vi "Sig_Digital_GetAttributes.vi"(0 "reference in":refnum<class "Sig_Digital.lvclass">, 1 "return data? (T)":bool=TRUE, 5 "error in (no error)":errorcluster) -> (14 "reference out":refnum<class "Sig_Digital.lvclass">, 15 "attributes ref":T3, 16 "attributes":T1, 19 "error out":errorcluster)   [LabVIEW 2019]
doc: "Returns a reference and if wanted the actual data values of the attributes. This method is used by the subclasses to access parent attributes."
uses:
  protected/ObjectAttributes.ctl
  Sig_Digital.lvclass
  ObjectAttributesRef.ctl
  <vilib>/addons/_AddQ/G#Object/G#Object.lvclass
  D:/LabASF/LabASF/src/Signal_class/Signal.lvclass
  D:/LabASF/LabASF/src/Proccess_class/Proccess.lvclass
  TypeDef/Config_Digital.ctl
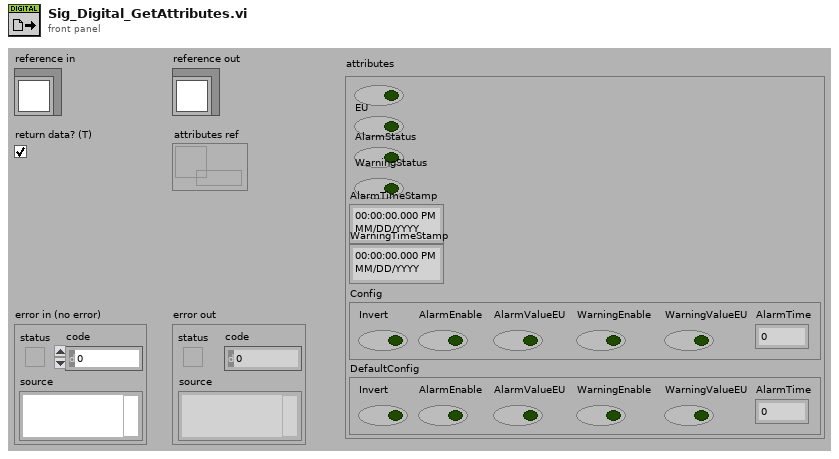
[diagram p1: front panel]
types:
  T1 = typedef "Sig_Digital.lvclass/ObjectAttributes.ctl" = cluster{"RAW":bool, "EU":bool, "AlarmStatus":bool, "WarningStatus":bool, "AlarmTimeStamp":timestamp, "WarningTimeStamp":timestamp, "Config":T2, "DefaultConfig":T2}
  T2 = typedef "Config_Digital.ctl" = cluster{"Invert":bool, "AlarmEnable":bool, "AlarmValueEU":bool, "WarningEnable":bool, "WarningValueEU":bool, "AlarmTime":dbl}
  T3 = typedef "Sig_Digital.lvclass/ObjectAttributesRef.ctl" = refnum<data-value>
  T4 = typedef "Sig_Digital.lvclass/ObjectAttributes.ctl" = cluster{}
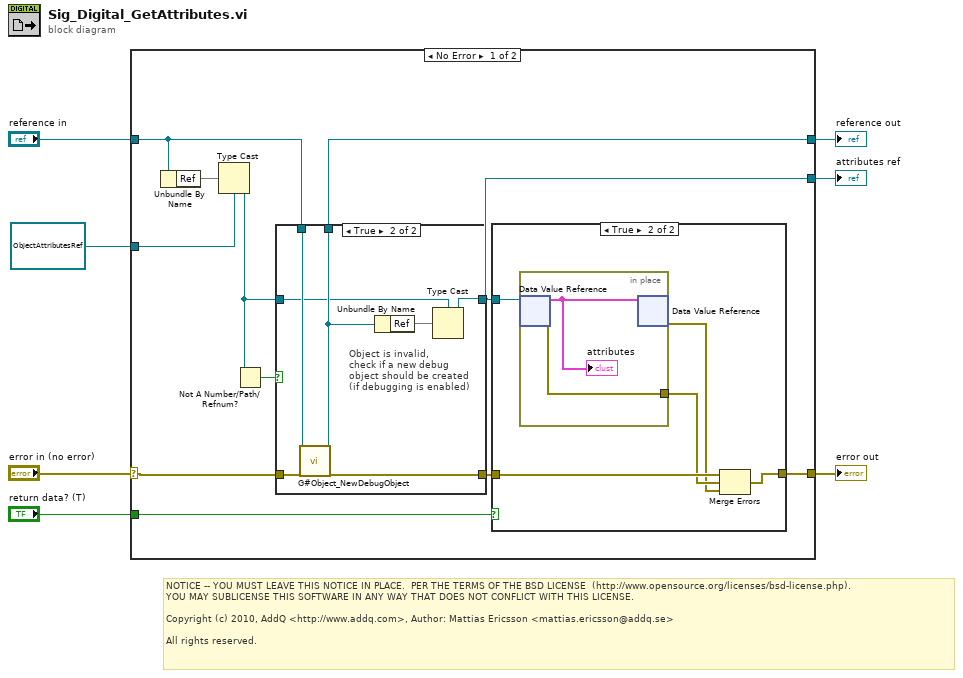
[diagram p0: block diagram]
diagram:
  # "NOTICE -- YOU MUST LEAVE THIS NOTICE IN PLACE.  PER THE TERMS OF THE BSD LICENSE  (http://www.opensource.org/licenses/bsd-license.php).\nYOU MAY SUBLICENSE THIS SOFTWARE IN ANY WAY THAT DOES NOT CONFLICT WITH THIS LICENSE.\n\nCopyright (c) 2010, AddQ <http://www.addq.com>, Author: Mattias Ericsson <mattias.ericsson@addq.se>\n\nAll rights reserved."
  n1 = case shown="No Error" "error in (no error)" {
    selector: "error in (no error)" -> [w14 w39]
    tunnel: [w17 w39] -> w6
    tunnel: [w11 w38] -> w4
    tunnel: "reference in" -> [w12 w38]
    tunnel: [w8 w37] -> w3
    tunnel: "return data? (T)" -> [w18 _]
    tunnel: T3 refnum ("attributes ref") -> [w10 w37]
    frame No Error {
      n2 = Unbundle By Name(w12) -> ("Ref"=w16)
      n3 = Type Cast(type=w10, x=w16) -> (*(type *) &x=w9:T3)
      n4 = Not A Number/Path/Refnum?(number/path/refnum=w9) -> (NaN/Path/Refnum?=w13:bool)
      n5 = case shown="True" w13 {
        tunnel: [w21 w28] -> w15
        tunnel: w14 -> [w21 w27]
        tunnel: w12 -> [w20 w26]
        tunnel: [w20 w24] -> w11
        tunnel: w9 -> [w19 w23]
        tunnel: [w19 w22] -> w8
        frame False {
        }
        frame True {
          # "Object is invalid,\ncheck if a new debug\nobject should be created\n(if debugging is enabled)"
          n6 = call <vilib>:"G#Object_NewDebugObject.vi"("reference in"=w26, "error in (no error)"=w27) -> ("reference out"=w24:refnum<class "G#Object.lvclass">, "error out"=w28:errorcluster)  [unwired: 16 in]
          n7 = Unbundle By Name(w24) -> ("Ref"=w25)
          n8 = Type Cast(type=w23, x=w25) -> (*(type *) &x=w22:T3)
        }
      }
      n9 = case shown="True" w18 {
        tunnel: w8 -> [_ w34]
        tunnel: w15 -> [w29 w33]
        tunnel: [w29 w32] -> w17
        frame False {
        }
        frame True {
          n10 = in-place {
            in-place-border: [w36] -> w31
            n11 = in-place-dvr #1(w34) -> (w35:T4, w36:errorcluster)
            "attributes" <- w35
            n12 = in-place-dvr #1(w35) -> (w30:errorcluster)  [unwired: 1 out]
          }
          n13 = Merge Errors(w33, w31, w30) -> (w32:errorcluster)
        }
      }
    }
    frame Error {
    }
  }
  "error out" <- w6
  "reference out" <- w4
  "attributes ref" <- w3
